vi "NT Read Multiple Entries as Generic.vi"(11 "Name Pattern":string) -> (0 "Success":bool, 2 "Names":string[](array[string]), 3 "Field Values":T1[](array[typedef]))   [LabVIEW 2017]
doc: "Return an array of tagged cluster data and ans array of names for the entries that match the name pattern. Supported wildcards are * and ?."
uses:
  <vilib>/Rock Robotics/Network Tables/Field Data.ctl
  <vilib>/Rock Robotics/Network Tables/Field Type.ctl
  <vilib>/Rock Robotics/Network Tables/Sequence.ctl
  <vilib>/Rock Robotics/Network Tables/Make Table Operation.ctl
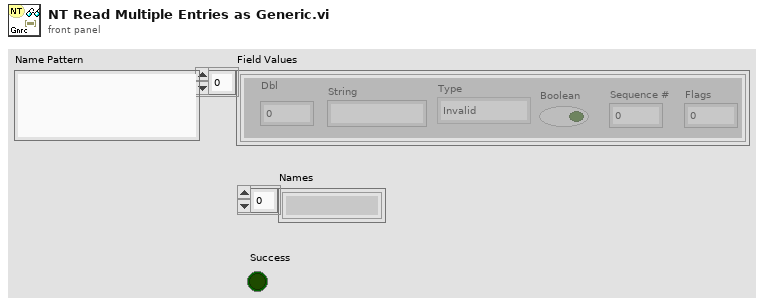
[diagram p1: front panel]
types:
  T1 = typedef "Field Data.ctl" = cluster{"Dbl":dbl, "String":string, "Type":T2, "Boolean":bool, "Sequence #":T3, "Flags":u8}
  T2 = typedef "Field Type.ctl" = enum8{"Invalid", "Bool", "Numeric", "String", "Raw", "Boolean Array", "Numeric Array", "String Array", "RPC"}
  T3 = typedef "Sequence.ctl" = u16
  T4 = typedef "Make Table Operation.ctl" = enum16{"Get or Add Field", "Get Field or Add Temp", "Replace Temp ID", "Get Field ID - No Add", "Get Table Field IDs", "Get Field ID Info", "Move Field to Temp", "Validate", "Remove Field", "Remove All"}
  T5 = typedef "Field ID.ctl" = i32
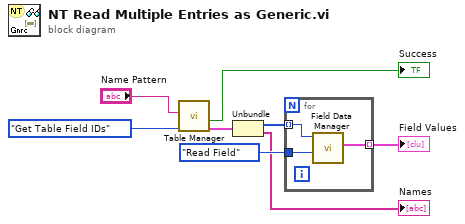
[diagram p0: block diagram]
diagram:
  n1 = call <vilib>:"Table Manager.vi"("Operation"=Make_Table_Operation."Get Table Field IDs", "Entry Name"="Name Pattern") -> ("Entries"=w3:cluster{"Entry IDs":T5[], "Names":string[]}, "Success"=→"Success":bool)  [unwired: 6 in, 2 out]
  n2 = Unbundle(w3) -> ("Entry IDs"=w2:T5[], "Names"=→"Names":string[])
  n3 = for {
    tunnel: [w11] -> w7 mode=indexing
    tunnel: w2 -> [w10] mode=indexing
    tunnel: enum16{"Update Field", "Read Field"}."Read Field" ("Operation") -> [w9]
    n4 = call <vilib>:"Field Data Manager.vi"("Operation"=w9, "Field ID"=w10) -> ("Field Value Out"=w11:T1)  [unwired: 8 in, 1 out]
  }
  "Field Values" <- w7
